vi "运维调试_综合生物毒性2.vi"() -> ()   [LabVIEW 2016, in "综合生物毒性.lvlib"]
uses:
  <vilib>/Plasmionique/MB Master/MB_Master_Serial/MB_Master_Serial.lvclass
  C:/Program Files (x86)/National Instruments/LabVIEW 2016/vi.lib/Plasmionique/MB Master/MB_Master/MB_Master.lvclass
  <vilib>/Plasmionique/MB Master/MB_Master/MB_Master.lvclass
  <vilib>/Plasmionique/MB Master/MB Master.lvlib
  <vilib>/ptbypt/NI_PtbyPt.lvlib
  <vilib>/Utility/config.llb/NI_LVConfig.lvlib
panel:
  out "工作中":bool
  out "存数据":bool
  in  "计数":u32
  out "标签.文本":string
  out "停止":bool
  out "自动清洗启动":bool
  out "自动复苏启动":bool
  out "纯水测量启动":bool
  out "质控测量启动":bool
  out "水样测量启动":bool
  in  "启动自动清洗":bool
  in  "启动自动复苏":bool
  in  "启动纯水测量":bool
  in  "启动质控测量":bool
  out "串口号":string
  out "通讯时长":string
  out "通讯":bool
  in  "参数设置":bool
  out "试剂余量":u32
  out "CF":sgl format="%#.6f"
  in  "综合生物毒性":bool=TRUE
  out "seconds current":timestamp
  out "seconds record":timestamp
  out "培养仓温度":sgl format="%#.2f ℃"
  out "简易步骤名称":string
  out "固件版本号":string
  out "模块版本号":string
  out "质控测量结果":sgl format="%#.2f"
  out "水样测量结果":sgl format="%#.2f "
  out "测量仓温度":sgl format="%#.2f ℃"
  out "St":i32
  out "Rt":i32
  out "S0":i32
  out "R0":i32
  out "运行状态":T1 {"数据时间:" format="%<%y/%m/%d %H:%M:%S>T"; "仪器时间:" format="%<%y/%m/%d %H:%M:%S>T"}
  out "集成报警信息":string
  in  "停止":bool
  in  "启动水样测量":bool
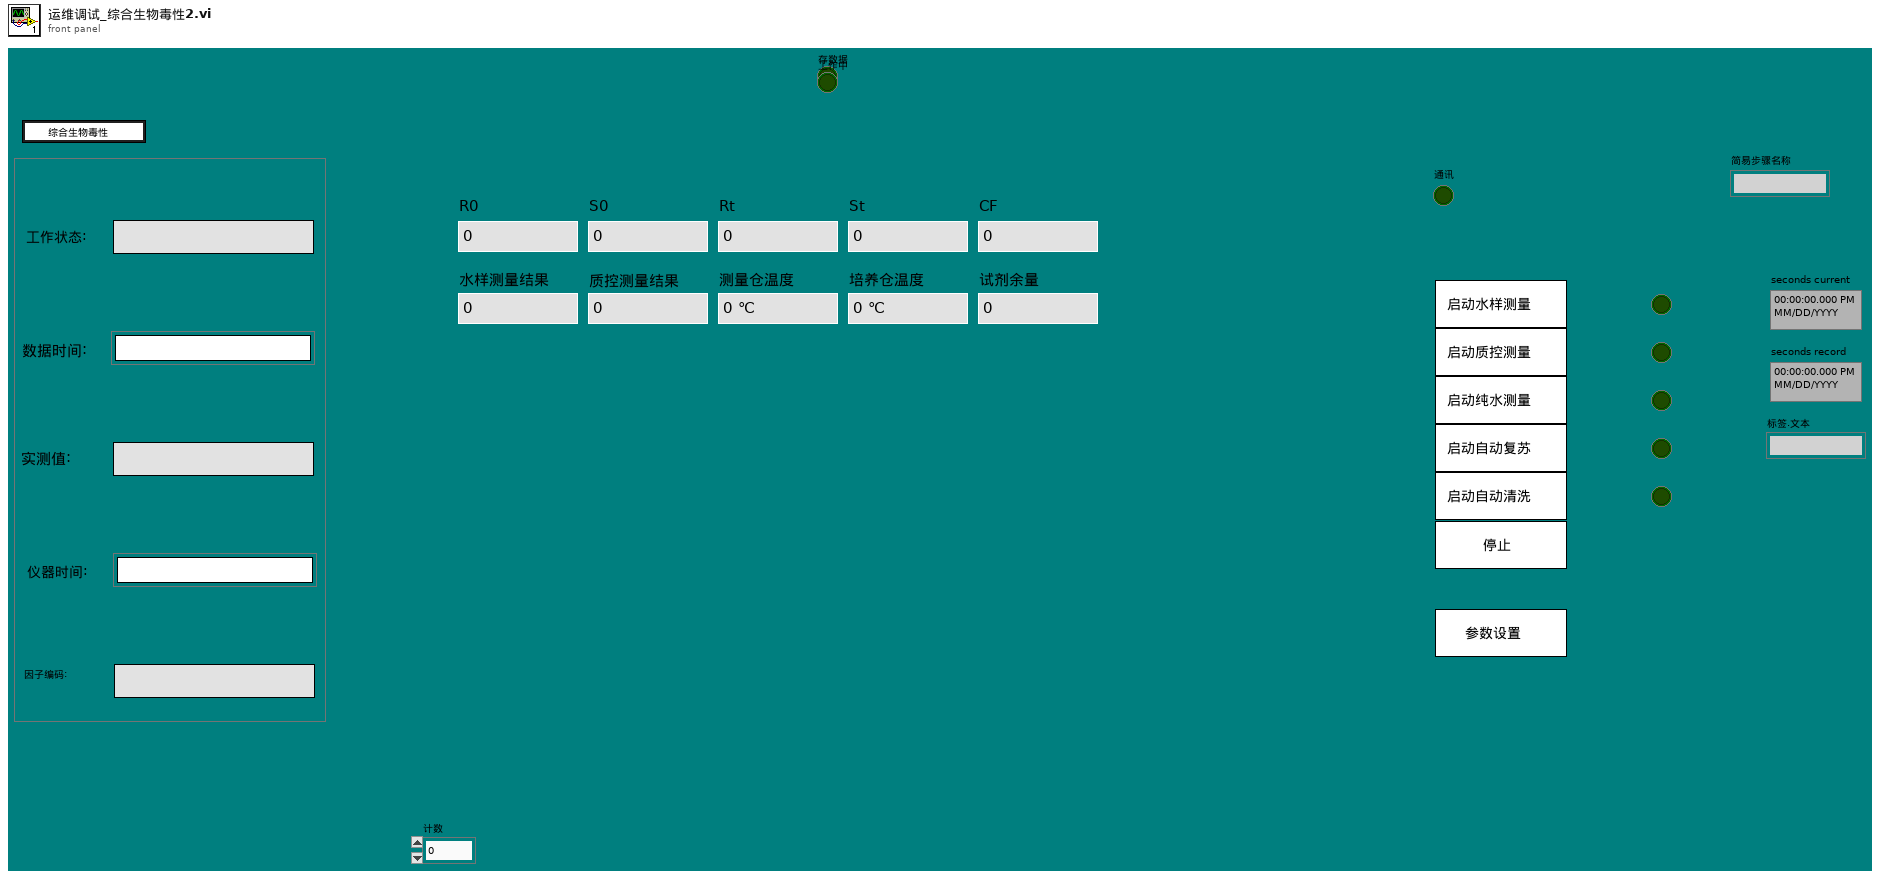
[diagram p1: front panel]
types:
  T1 = cluster{"工作状态:":string, "数据时间:":timestamp, "实测值:":string, "仪器时间:":timestamp, "因子编码:":string}
  T2 = cluster{"Major":u16, "Minor":u16, "Fix":u16, "Build":u16}
  T3 = typedef "NI_LVConfig.lvlib/Config Data RefNum.ctl" = refnum<k1>
  T4 = enum8{"Enabled", "Disabled", "Disabled and Grayed Out"}
  T5 = cluster{"baud rate (bps)":u32, "stop bits":u16, "parity":u16, "flow control":u16, "timeout":u32, "retries":i32}
  T6 = cluster{"时间":timestamp, "水样测量结果":sgl, "质控测量结果":sgl, "R0":i32, "S0":i32, "Rt":i32, "St":i32, "CF":sgl, "测量仓温度":sgl, "培养仓温度":sgl, "试剂余量":u32, "仪器状态":string, "空白结果":dbl, "启动测量":enum32{"无", "启动水样测量", "启动质控测量", "启动纯水测量", "启动自动复苏", "启动自动清洗"}, "停止测量":bool}
  T7 = enum8{"Enabled", "Disabled", "Disabled and Grayed Out"}[]
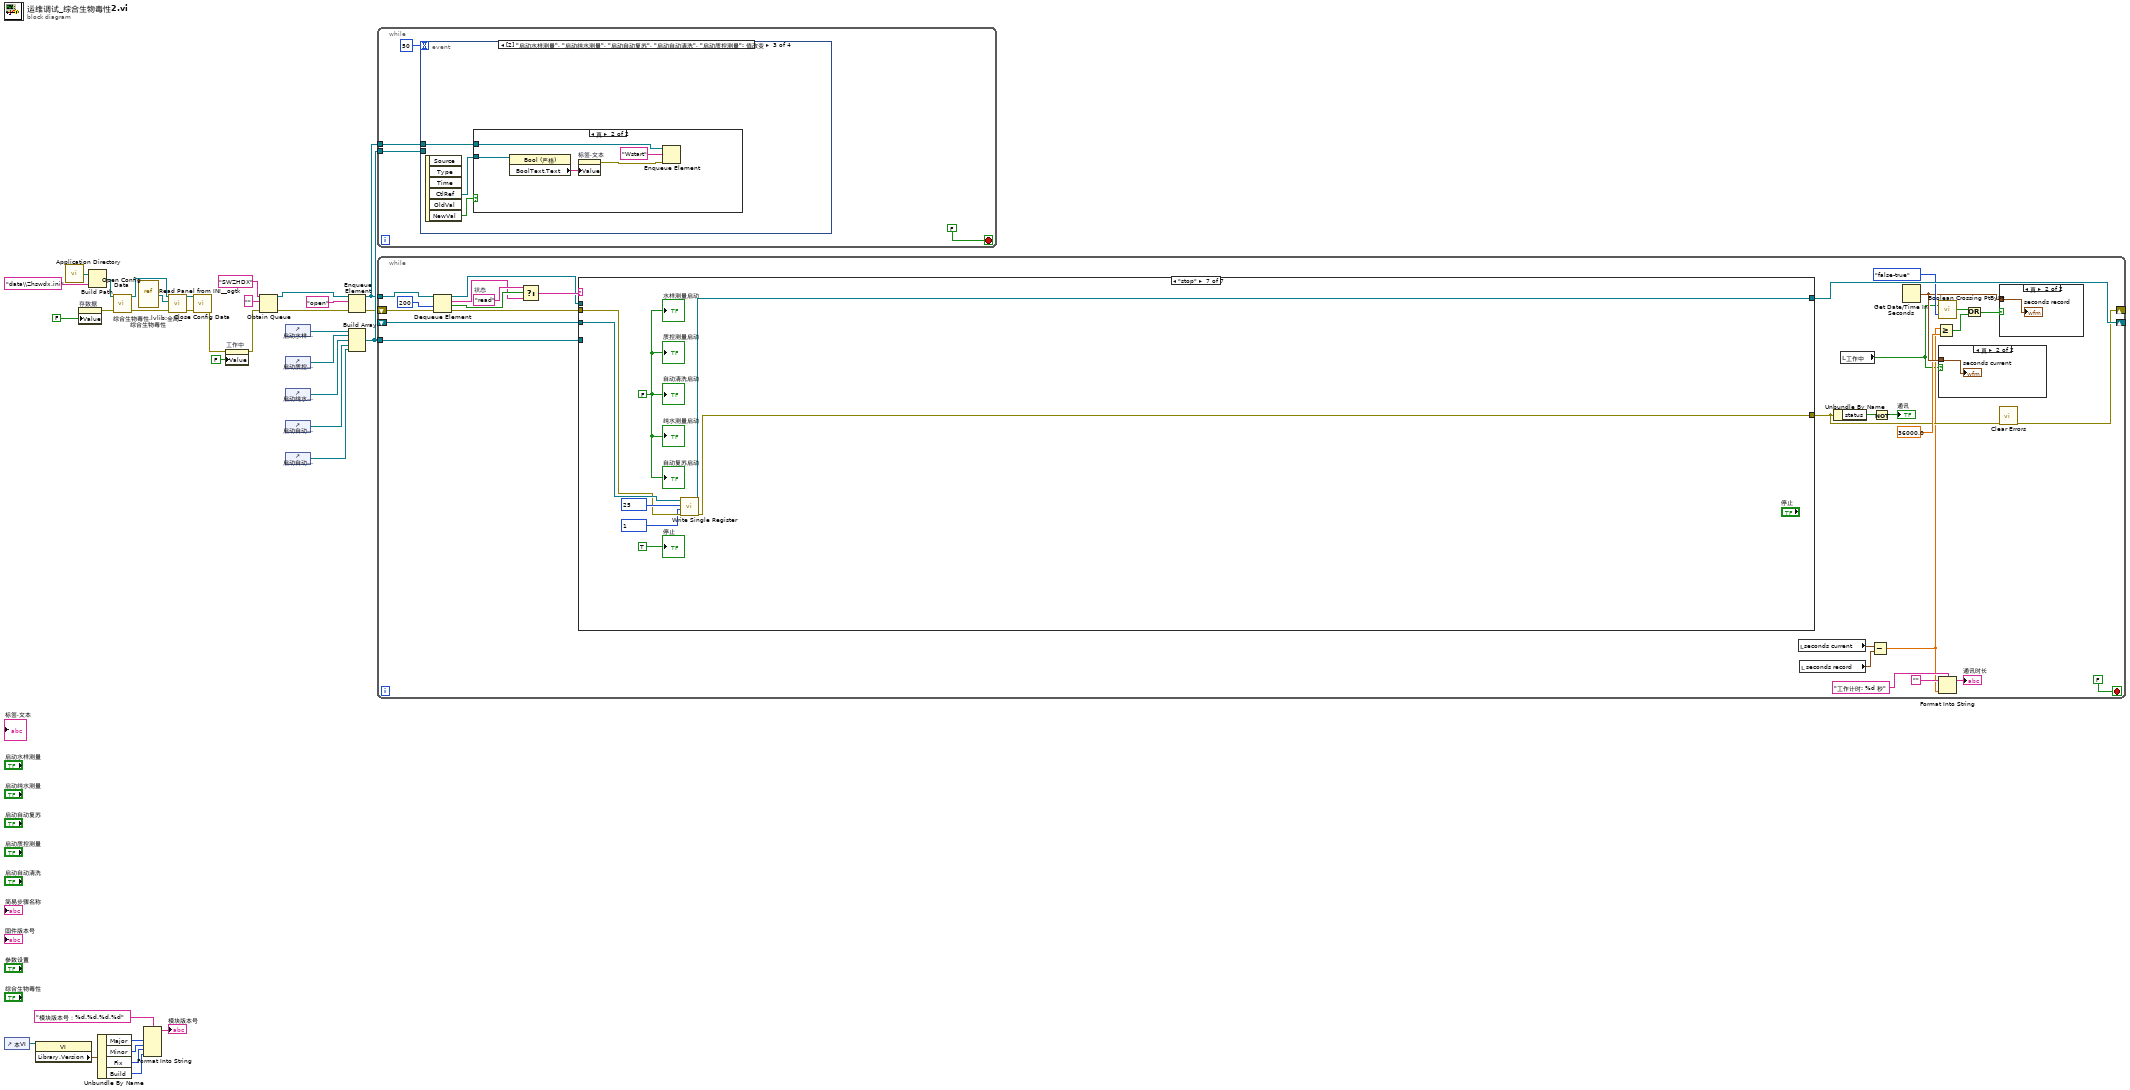
[diagram p0: block diagram]
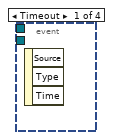
[diagram p2: hidden frame]
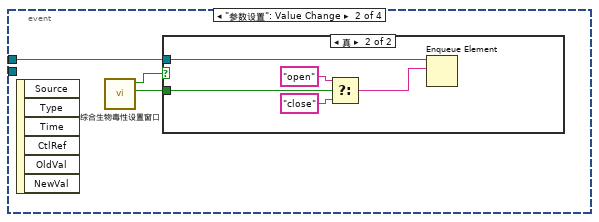
[diagram p3: hidden frame]
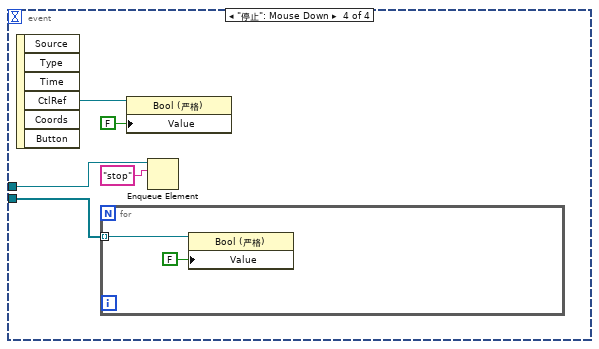
[diagram p6: hidden frame]
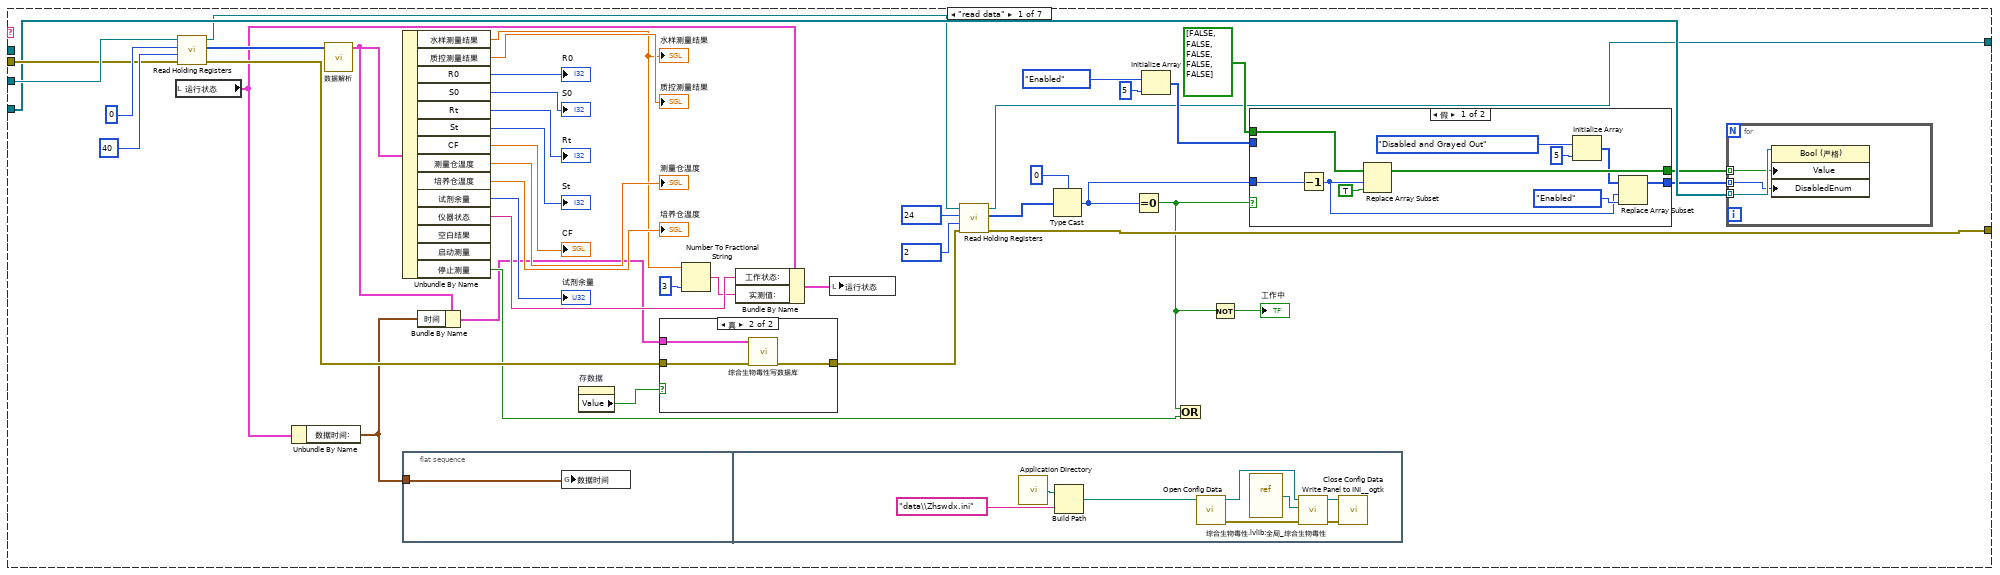
[diagram p9: hidden frame]
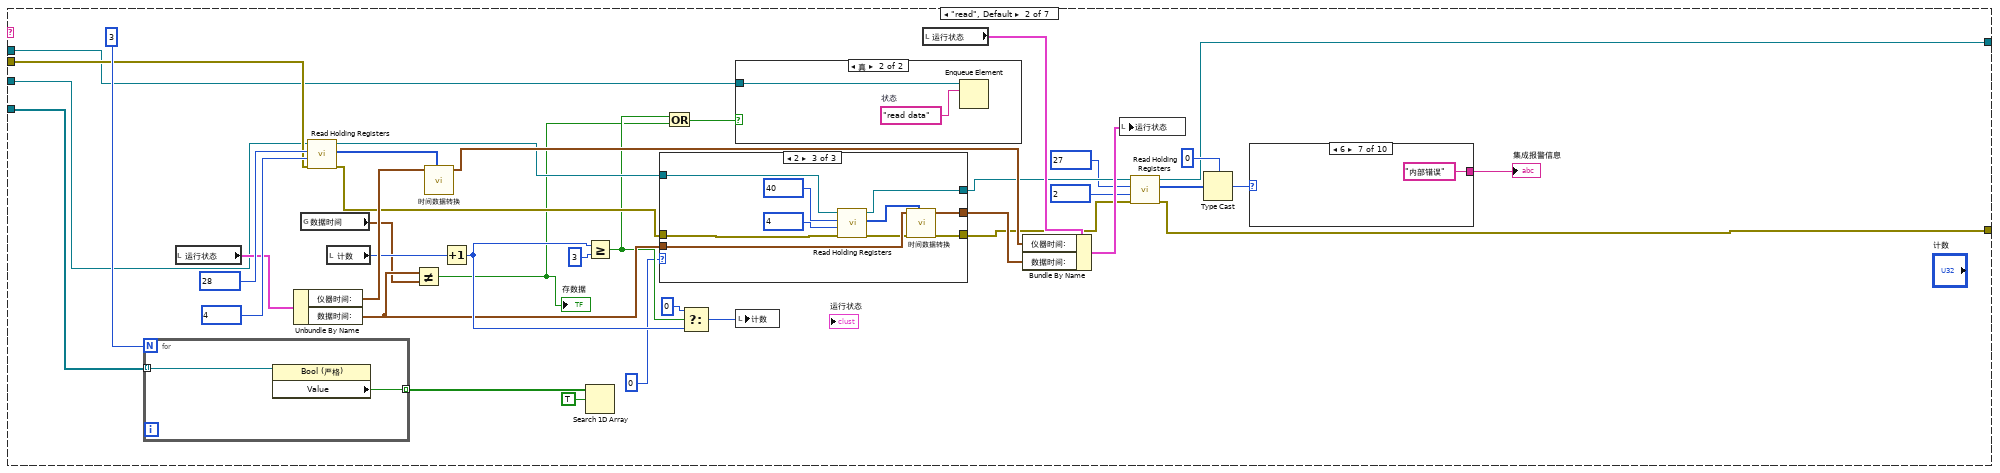
[diagram p12: hidden frame]
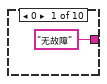
[diagram p13: hidden frame]
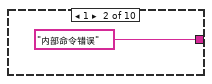
[diagram p14: hidden frame]
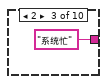
[diagram p15: hidden frame]
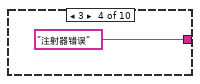
[diagram p16: hidden frame]
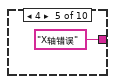
[diagram p17: hidden frame]
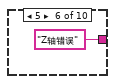
[diagram p18: hidden frame]
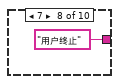
[diagram p19: hidden frame]
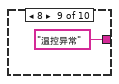
[diagram p20: hidden frame]
diagram:
  n1 = control-ref of="本VI"() -> (w34:refnum<vi>)
  n2 = property class="VI"(reference=w34) -> ("Library.Version"=w33:T2)  [unwired: 1 in, 2 out]
  n3 = call <vilib>:"Application Directory.vi"() -> ("Application Directory"=w20:path)
  n4 = property on="存数据" class="Bool (严格)"("Value"=FALSE ("存数据")) -> (error out=w4:errorcluster)  [unwired: 2 in, 1 out]
  n5 = Build Path(base path=w20, name or relative path="data\\Zhswdx.ini" ("名称或相对路径")) -> (appended path=w22:path)
  n6 = Unbundle By Name(w33) -> ("Major"=w31:u16, "Minor"=w30:u16, "Fix"=w29:u16, "Build"=w28:u16)
  n7 = call <vilib>:"Open Config Data.vi"("error in (no error)"=w4, "configuration file path"=w22) -> ("error out"=w18:errorcluster, "refnum"=w23:T3)  [unwired: 7 in, 1 out]
  n8 = vi-ref "综合生物毒性.lvlib:全局_综合生物毒性.vi"() -> (w17:refnum<vi>)
  n9 = Format Into String(format string="模块版本号：%d.%d.%d.%d" ("格式字符串"), w31, w30, w29, w28) -> (resulting string=→"模块版本号":string)  [unwired: 2 in, 1 out]
  n10 = call <userlib>:"Read Panel from INI__ogtk.vi"("error in (no error)"=w18, "VI ref"=w17, "refnum"=w23) -> ("error out"=w19:errorcluster, "refnum out"=w24:T3)  [unwired: 7 in]
  n11 = call <vilib>:"Close Config Data.vi"("error in (no error)"=w19, "refnum"=w24) -> ("error out"=w2:errorcluster)  [unwired: 8 in, 1 out]
  n12 = property on="工作中" class="Bool (严格)"(error in=w2, "Value"=FALSE ("工作中")) -> (error out=w1:errorcluster)  [unwired: 1 in, 1 out]
  n13 = Obtain Queue(name (unnamed)="SWZHDX" ("名称（未命名）"), element data type="" ("状态"), error in (no error)=w1) -> (queue out=w11:refnum<queue>, error out=w10:errorcluster)  [unwired: 2 in, 1 out]
  n14 = control-ref of="启动水样测量"() -> (w6:refnum<vi>)
  n15 = control-ref of="启动质控测量"() -> (w16:refnum<vi>)
  n16 = control-ref of="启动纯水测量"() -> (w15:refnum<vi>)
  n17 = control-ref of="启动自动复苏"() -> (w14:refnum<vi>)
  n18 = control-ref of="启动自动清洗"() -> (w13:refnum<vi>)
  n19 = Enqueue Element(queue=w11, element="open" ("状态"), error in (no error)=w10) -> (queue out=w8:refnum<queue>, error out=w7:errorcluster)  [unwired: 1 in, 1 out]
  n20 = Build Array(w6, w16, w15, w14, w13) -> (w12:refnum<vi>[])
  n21 = while {
    tunnel: w8 -> [w36]
    tunnel: w12 -> [w35]
    stop <- FALSE stop-if-true
    n22 = event shown="[2] \"启动水样测量\", \"启动纯水测量\", \"启动自动复苏\", \"启动自动清洗\", \"启动质控测量\": 值改变" {
      selector: _ -> [_ _ _ _]
      dyn-events: _ -> [_ _ _ _]
      timeout: 50 -> [_ _ _ _]
      tunnel: w36 -> [_ w39 w49 w59]
      tunnel: w35 -> [_ _ _ w55]
      event Timeout {
        n23 = event-data() -> ()  [unwired: 1 in, 3 out]
      }
      event "参数设置": Value Change {
        n24 = event-data() -> ()  [unwired: 1 in, 6 out]
        n25 = call "综合生物毒性设置窗口.vi"() -> ("开关"=w40:bool, "确定输出"=w41:bool)  [unwired: 10 in]
        n26 = case shown="真" w41 {
          tunnel: w40 -> [_ w46]
          tunnel: w39 -> [_ w42]
          frame False {
          }
          frame True {
            n27 = Select(t="open" ("状态"), s=w46, f="close" ("状态")) -> (s? t:f=w43:string)
            n28 = Enqueue Element(queue=w42, element=w43) -> ()  [unwired: 2 in, 3 out]
          }
        }
      }
      event "启动水样测量", "启动纯水测量", "启动自动复苏", "启动自动清洗", "启动质控测量": Value Change {
        n29 = event-data() -> ("CtlRef"=w47:refnum<vi>, "NewVal"=w48:bool)  [unwired: 1 in, 4 out]
        n30 = case shown="真" w48 {
          tunnel: w49 -> [_ w54]
          tunnel: w47 -> [_ w52]
          frame False {
          }
          frame True {
            n31 = property class="Bool (严格)"(reference=w52) -> ("BoolText.Text"=w51:string)  [unwired: 1 in, 2 out]
            n32 = property on="标签.文本" class="Str"("Value"=w51) -> (error out=w50:errorcluster)  [unwired: 2 in, 1 out]
            n33 = Enqueue Element(queue=w54, element="Wstart" ("元素"), error in (no error)=w50) -> ()  [unwired: 1 in, 3 out]
          }
        }
      }
      event "停止": Mouse Down {
        n34 = event-data() -> ("CtlRef"=w57:refnum<vi>)  [unwired: 1 in, 5 out]
        n35 = for {
          tunnel: w55 -> [w61] mode=indexing
          n36 = property class="Bool (严格)"(reference=w61, "Value"=FALSE ("值")) -> ()  [unwired: 1 in, 2 out]
        }
        n37 = property class="Bool (严格)"(reference=w57, "Value"=FALSE ("值")) -> ()  [unwired: 1 in, 2 out]
        n38 = Enqueue Element(queue=w59, element="stop" ("元素")) -> ()  [unwired: 2 in, 3 out]
      }
    }
  }
  n39 = while {
    shift-right: [w91] -> _
    shift-left: _ -> [w90]
    shift-right: [w68] -> _
    shift-left: w7 -> [w65]
    tunnel: w8 -> [w87]
    tunnel: w12 -> [w70]
    stop <- FALSE stop-if-true
    w84 = "read"  # 状态
    n40 = Dequeue Element(queue=w87, timeout in ms (-1)=200 ("超时毫秒(-1)"), error in (no error)=w65) -> (queue out=w66:refnum<queue>, element=w83:string, timed out?=w85:bool, error out=w64:errorcluster)
    n41 = Select(t=w84, s=w85, f=w83) -> (s? t:f=w67:string)
    n42 = case shown="\"stop\"" w67 {
      tunnel: [w103 w169 w258 w268 w281 w301 w303] -> w91
      tunnel: w90 -> [w137 w190 _ w268 w280 w300 w309]
      tunnel: w64 -> [w125 w191 _ w270 w278 w298 w307]
      tunnel: [w101 w167 w257 w269 w274 w297 w302] -> w69
      tunnel: w70 -> [w122 w197 _ _ w272 _ _]
      tunnel: w66 -> [_ w187 _ _ _ _ _]
      frame "read data" {
        n43 = local read "运行状态"() -> (w99:T1)
        n44 = call <vilib>:"Read Holding Registers.vi"("error in (no error)"=w125, "quantity"=u16 40, "starting address"=u16 0, "MB session in"=w137) -> ("error out"=w124:errorcluster, "Registers"=w121:u16[], "MB session out"=w104:refnum<class "MB_Master.lvclass">)  [unwired: 5 in]
        n45 = Unbundle By Name(w99) -> ("数据时间:"=w97:timestamp)
        n46 = call "数据解析.vi"("数组"=w121) -> ("综合生物毒性"=w98:T6)  [unwired: 9 in, 1 out]
        n47 = Unbundle By Name(w98) -> ("水样测量结果"=w118:sgl, "质控测量结果"=→"质控测量结果":sgl, "R0"=→"R0":i32, "S0"=→"S0":i32, "Rt"=→"Rt":i32, "St"=→"St":i32, "CF"=→"CF":sgl, "测量仓温度"=→"测量仓温度":sgl, "培养仓温度"=→"培养仓温度":sgl, "试剂余量"=→"试剂余量":u32, "仪器状态"=w120:string, "停止测量"=w123:bool)  [unwired: 2 out]
        "水样测量结果" <- w118
        n48 = flat-sequence {
          tunnel: w97 -> [w138]
          frame #0 {
            n49 = global write "全局_综合生物毒性.vi" "数据时间"(w138) -> ()
          }
          frame #1 {
            n50 = call <vilib>:"Application Directory.vi"() -> ("Application Directory"=w143:path)
            n51 = Build Path(base path=w143, name or relative path="data\\Zhswdx.ini" ("名称或相对路径")) -> (appended path=w141:path)
            n52 = call <vilib>:"Open Config Data.vi"("configuration file path"=w141) -> ("error out"=w145:errorcluster, "refnum"=w140:T3)  [unwired: 8 in, 1 out]
            n53 = vi-ref "综合生物毒性.lvlib:全局_综合生物毒性.vi"() -> (w146:refnum<vi>)
            n54 = call <userlib>:"Write Panel to INI__ogtk.vi"("error in (no error)"=w145, "VI ref"=w146, "refnum"=w140) -> ("error out"=w144:errorcluster, "refnum out"=w139:T3)  [unwired: 7 in]
            n55 = call <vilib>:"Close Config Data.vi"("error in (no error)"=w144, "refnum"=w139) -> ()  [unwired: 8 in, 2 out]
          }
        }
        n56 = Bundle By Name(cluster=w98, "时间"=w97) -> (w96:T6)
        n57 = property on="存数据" class="Bool (严格)"() -> ("Value"=w100:bool)  [unwired: 2 in, 2 out]
        n58 = case shown="真" w100 {
          tunnel: w96 -> [_ w165]
          tunnel: w124 -> [w162 w164]
          tunnel: [w162 w163] -> w102
          frame False {
          }
          frame True {
            n59 = call "综合生物毒性写数据库.vi"("错误输入（无错误）"=w164, "综合生物毒性"=w165) -> ("错误输出"=w163:errorcluster)  [unwired: 9 in]
          }
        }
        n60 = Number To Fractional String(number=w118, precision (6)=i16 3 ("精度(6)")) -> (F-format string=w116:string)  [unwired: 2 in]
        n61 = Bundle By Name(cluster=w99, "工作状态:"=w120, "实测值:"=w116) -> (w119:T1)
        n62 = local write "运行状态"(w119) -> ()
        n63 = call <vilib>:"Read Holding Registers.vi"("error in (no error)"=w102, "quantity"=u16 2 ("starting address"), "starting address"=u16 24, "MB session in"=w104) -> ("error out"=w101:errorcluster, "Registers"=w106:u16[], "MB session out"=w103:refnum<class "MB_Master.lvclass">)  [unwired: 5 in]
        n64 = Type Cast(type=u32 0 ("数字"), x=w106) -> (*(type *) &x=w105:u32)
        n65 = Equal To 0?(x=w105) -> (x = 0?=w95:bool)
        n66 = Initialize Array(T4."Enabled" ("禁用"), 5 ("维数大小")) -> (w111:T7)
        n67 = Or(x=w95, y=w123) -> ()  [unwired: 1 out]
        n68 = Not(x=w95) -> (.not. x?=→"工作中":bool)
        n69 = case shown="假" w95 {
          tunnel: bool[] [FALSE, FALSE, FALSE, FALSE, FALSE] -> [w159 w161]
          tunnel: [w156 w161] -> w114
          tunnel: w105 -> [w158 _]
          tunnel: w111 -> [_ w160]
          tunnel: [w150 w160] -> w110
          frame False {
            n70 = Decrement(x=w158) -> (x-1=w151:u32)
            n71 = Replace Array Subset(array=w159, new element=TRUE ("新元素/子数组"), index=w151) -> (w156:bool[])
            n72 = Initialize Array(T4."Disabled and Grayed Out" ("禁用"), 5 ("维数大小")) -> (w152:T7)
            n73 = Replace Array Subset(array=w152, new element=T4."Enabled" ("禁用"), index=w151) -> (w150:T7)
          }
          frame True {
          }
        }
        n74 = for {
          tunnel: w122 -> [w149] mode=indexing
          tunnel: w114 -> [w148] mode=indexing
          tunnel: w110 -> [w147] mode=indexing
          n75 = property class="Bool (严格)"(reference=w149, "Value"=w148, "DisabledEnum"=w147) -> ()  [unwired: 1 in, 2 out]
        }
      }
      frame "read", Default {
        n76 = for {
          N: 3 -> [_]
          tunnel: w197 -> [w248] mode=indexing
          tunnel: [w247] -> w195 mode=indexing
          n77 = property class="Bool (严格)"(reference=w248) -> ("Value"=w247:bool)  [unwired: 1 in, 2 out]
        }
        n78 = local read "运行状态"() -> (w200:T1)
        n79 = Unbundle By Name(w200) -> ("仪器时间:"=w199:timestamp, "数据时间:"=w181:timestamp)
        n80 = global read "全局_综合生物毒性.vi" "数据时间"() -> (w180:timestamp)
        n81 = call <vilib>:"Read Holding Registers.vi"("error in (no error)"=w191, "quantity"=u16 4 ("starting address"), "starting address"=u16 28, "MB session in"=w190) -> ("error out"=w188:errorcluster, "Registers"=w201:u16[], "MB session out"=w189:refnum<class "MB_Master.lvclass">)  [unwired: 5 in]
        n82 = local read "计数"() -> (w186:u32)
        n83 = Not Equal?(x=w181, y=w180) -> (x != y?=w178:bool)
        "存数据" <- w178
        n84 = call "时间数据转换.vi"("时间寄存器"=w201, "时间"=w199) -> ("time stamp"=w198:timestamp)  [unwired: 8 in, 1 out]
        n85 = Increment(x=w186) -> (x+1=w184:u32)
        n86 = Greater Or Equal?(x=w184, y=u32 3) -> (x >= y?=w179:bool)
        n87 = Search 1D Array(1D array=w195, element=TRUE ("元素")) -> ()  [unwired: 1 in, 1 out]
        n88 = case shown="2" 0 ("index of element") {
          tunnel: w189 -> [w224 w234 w244]
          tunnel: w181 -> [w222 w232 w242]
          tunnel: [w221 w231 w241] -> w193
          tunnel: w188 -> [w220 w227 w240]
          tunnel: [w218 w230 w237] -> w176
          tunnel: [w217 w228 w238] -> w168
          frame 0, Default {
            n89 = call <vilib>:"Read Holding Registers.vi"("error in (no error)"=w220, "quantity"=u16 4 ("starting address"), "starting address"=u16 32, "MB session in"=w224) -> ("error out"=w219:errorcluster, "Registers"=w223:u16[], "MB session out"=w218:refnum<class "MB_Master.lvclass">)  [unwired: 5 in]
            n90 = call "时间数据转换.vi"("时间寄存器"=w223, "error in (no error)"=w219, "时间"=w222) -> ("error out"=w217:errorcluster, "time stamp"=w221:timestamp)  [unwired: 7 in]
          }
          frame 1 {
            n91 = call <vilib>:"Read Holding Registers.vi"("error in (no error)"=w227, "quantity"=u16 4 ("starting address"), "starting address"=u16 36, "MB session in"=w234) -> ("error out"=w229:errorcluster, "Registers"=w233:u16[], "MB session out"=w230:refnum<class "MB_Master.lvclass">)  [unwired: 5 in]
            n92 = call "时间数据转换.vi"("时间寄存器"=w233, "error in (no error)"=w229, "时间"=w232) -> ("error out"=w228:errorcluster, "time stamp"=w231:timestamp)  [unwired: 7 in]
          }
          frame 2 {
            n93 = call <vilib>:"Read Holding Registers.vi"("error in (no error)"=w240, "quantity"=u16 4 ("starting address"), "starting address"=u16 40, "MB session in"=w244) -> ("error out"=w239:errorcluster, "Registers"=w243:u16[], "MB session out"=w237:refnum<class "MB_Master.lvclass">)  [unwired: 5 in]
            n94 = call "时间数据转换.vi"("时间寄存器"=w243, "error in (no error)"=w239, "时间"=w242) -> ("error out"=w238:errorcluster, "time stamp"=w241:timestamp)  [unwired: 7 in]
          }
        }
        n95 = Or(x=w179, y=w178) -> (x .or. y?=w177:bool)
        n96 = Select(t=u32 0, s=w179, f=w184) -> (s? t:f=w182:u32)
        n97 = case shown="真" w177 {
          tunnel: w187 -> [_ w216]
          frame False {
          }
          frame True {
            w215 = "read data"  # 状态
            n98 = Enqueue Element(queue=w216, element=w215) -> ()  [unwired: 2 in, 3 out]
          }
        }
        n99 = local write "计数"(w182) -> ()
        n100 = local read "运行状态"() -> (w202:T1)
        n101 = Bundle By Name(cluster=w202, "仪器时间:"=w198, "数据时间:"=w193) -> (w192:T1)
        n102 = local write "运行状态"(w192) -> ()
        n103 = call <vilib>:"Read Holding Registers.vi"("error in (no error)"=w168, "quantity"=u16 2 ("starting address"), "starting address"=u16 27, "MB session in"=w176) -> ("error out"=w167:errorcluster, "Registers"=w173:u16[], "MB session out"=w169:refnum<class "MB_Master.lvclass">)  [unwired: 5 in]
        n104 = Type Cast(type=0, x=w173) -> (*(type *) &x=w171:i32)
        n105 = case shown="6" w171 {
          tunnel: ["无故障" "内部命令错误" "系统忙" "注射器错误" "X轴错误" "Z轴错误" "内部错误" "用户终止" "温控异常" "未知错误"] -> w170
          frame 0 {
          }
          frame 1 {
          }
          frame 2 {
          }
          frame 3 {
          }
          frame 4 {
          }
          frame 5 {
          }
          frame 6 {
          }
          frame 7 {
          }
          frame 8 {
          }
          frame 9, Default {
          }
        }
        "集成报警信息" <- w170
      }
      frame "open" {
        n106 = global read "全局_综合生物毒性.vi" "VISA Resource"() -> (w264:refnum<visa-resource-name>)
        n107 = Type Cast(x=w264) -> (*(type *) &x=→"串口号":string)  [unwired: 1 in]
        n108 = call <vilib>:"Open Serial Session.vi"("Mode (RTU)"=enum16{"RTU", "ASCII"}."RTU", "Slave ID"=u8 1, "Serial Config"=T5 {"baud rate (bps)"=9600, "stop bits"=10, "parity"=0, "flow control"=0, "timeout"=2000, "retries"=1}, "VISA Resource"=w264) -> ("Error out"=w260:errorcluster, "MB_Serial session"=w259:refnum<class "MB_Master_Serial.lvclass">)  [unwired: 6 in]
        n109 = call <vilib>:"Read Holding Registers.vi"("error in (no error)"=w260, "quantity"=u16 2 ("starting address"), "starting address"=u16 26, "MB session in"=w259) -> ("error out"=w257:errorcluster, "Registers"=w255:u16[], "MB session out"=w258:refnum<class "MB_Master_Serial.lvclass">)  [unwired: 5 in]
        n110 = Type Cast(type=0, x=w255) -> (*(type *) &x=w252:i32)
        n111 = local read "运行状态"() -> (w251:T1)
        n112 = Format Into String(format string="%4d" ("格式字符串"), initial string="w0" ("初始字符串"), w252) -> (resulting string=w249:string)  [unwired: 1 in, 1 out]
        n113 = Bundle By Name(cluster=w251, "因子编码:"=w249) -> (w250:T1)
        n114 = local write "运行状态"(w250) -> ()
      }
      frame "close" {
        n115 = call-dynamic "Close Session.vi"("error in (no error)"=w270, "MB session in"=w268) -> ("error out"=w269:errorcluster)  [unwired: 9 in]
      }
      frame "Wstart" {
        n116 = for {
          tunnel: w272 -> [w283] mode=indexing
          tunnel: [w282] -> w271 mode=indexing
          n117 = property class="Bool (严格)"(reference=w283) -> ("BoolText.Text"=w282:string)  [unwired: 1 in, 2 out]
        }
        n118 = local read "标签.文本"() -> (w276:string)
        n119 = Search 1D Array(1D array=w271, element=w276) -> (index of element=w275:i32)  [unwired: 1 in]
        n120 = Increment(x=w275) -> (x+1=w277:i32)
        n121 = To Unsigned Word Integer(number=w277) -> (unsigned 16bit integer=w273:u16)
        n122 = call <vilib>:"Write Single Register.vi"("error in (no error)"=w278, "value"=w273, "address"=u16 24 ("starting address"), "MB session in"=w280) -> ("error out"=w274:errorcluster, "MB session out"=w281:refnum<class "MB_Master.lvclass">)  [unwired: 6 in]
        n123 = case shown="无错误" w274 {
          tunnel: w275 -> [w286 _]
          tunnel: w272 -> [w287 _]
          frame No Error {
            n124 = Index Array(array=w287, index=w286) -> (element=w284:refnum<vi>)
            n125 = control-ref of="水样测量启动"() -> (w295:refnum<vi>)
            n126 = control-ref of="质控测量启动"() -> (w294:refnum<vi>)
            n127 = control-ref of="自动清洗启动"() -> (w291:refnum<vi>)
            n128 = control-ref of="纯水测量启动"() -> (w293:refnum<vi>)
            n129 = control-ref of="自动复苏启动"() -> (w292:refnum<vi>)
            n130 = property class="Bool (严格)"(reference=w284, "Value"=TRUE ("值")) -> ()  [unwired: 1 in, 2 out]
            n131 = Build Array(w295, w294, w293, w292, w291) -> (w290:refnum<vi>[])
            n132 = Index Array(array=w290, index=w286) -> (element=w289:refnum<vi>)
            n133 = property class="Bool (严格)"(reference=w289, "Value"=TRUE ("值")) -> ()  [unwired: 1 in, 2 out]
          }
          frame Error {
          }
        }
      }
      frame "Qstart" {
        n134 = call <vilib>:"Write Single Register.vi"("error in (no error)"=w298, "value"=u16 2 ("starting address"), "address"=u16 24 ("starting address"), "MB session in"=w300) -> ("error out"=w297:errorcluster, "MB session out"=w301:refnum<class "MB_Master.lvclass">)  [unwired: 6 in]
      }
      frame "stop" {
        w304 = FALSE
        n135 = call <vilib>:"Write Single Register.vi"("error in (no error)"=w307, "value"=u16 1 ("starting address"), "address"=u16 25 ("starting address"), "MB session in"=w309) -> ("error out"=w302:errorcluster, "MB session out"=w303:refnum<class "MB_Master.lvclass">)  [unwired: 6 in]
        "自动清洗启动" <- w304
        "自动复苏启动" <- w304
        "停止" <- TRUE ("停止")
        "水样测量启动" <- w304
        "质控测量启动" <- w304
        "纯水测量启动" <- w304
      }
    }
    n136 = local read "seconds current"() -> (w79:timestamp)
    n137 = local read "seconds record"() -> (w78:timestamp)
    n138 = Unbundle By Name(w69) -> ("status"=w88:bool)
    n139 = local read "工作中"() -> (w62:bool)
    n140 = Subtract(x=w79, y=w78) -> (x-y=w63:dbl)
    n141 = Not(x=w88) -> (.not. x?=→"通讯":bool)
    n142 = Get Date/Time In Seconds() -> (seconds since 1Jan1904=w80:timestamp)
    n143 = Greater Or Equal?(x=w63, y=36000.0) -> (x >= y?=w75:bool)
    n144 = call <vilib>:"Boolean Crossing PtByPt.vi"("direction"=enum16{"either", "false-true", "true-false"}."false-true", "input"=w62) -> ("crossing"=w76:bool)  [unwired: 1 in]
    n145 = case shown="真" w62 {
      tunnel: w80 -> [_ w92]
      frame False {
      }
      frame True {
        "seconds current" <- w92
      }
    }
    n146 = Format Into String(format string="工作计时: %d 秒" ("格式字符串"), initial string="", w63) -> (resulting string=→"通讯时长":string)  [unwired: 1 in, 1 out]
    n147 = Or(x=w76, y=w75) -> (x .or. y?=w74:bool)
    n148 = case shown="真" w74 {
      tunnel: w80 -> [_ w93]
      frame False {
      }
      frame True {
        "seconds record" <- w93
      }
    }
    n149 = call <vilib>:"Clear Errors.vi"("error in (no error)"=w69) -> ("error out"=w68:errorcluster)  [unwired: 5 in, 1 out]
  }
